vi "AVQ8347 Span Span.vi"(8 "Error In":errorcluster, 9 "Span Unit (nm)":T1(ring)=enum."nm", 10 "Span Value (700)":dbl=700.0 format="%.2f", 11 "VISA Session":refnum<visa-resource-name>) -> (0 "Error Out":errorcluster, 2 "Send Code":string, 3 "Copy VISA Session":refnum<visa-resource-name>)   [LabVIEW 2018]
doc: "Setting of the analysis wavelength span"
panel:
  # "Span Span"
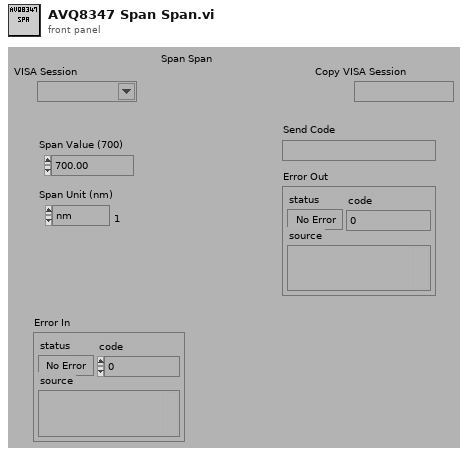
[diagram p1: front panel]
types:
  T1 = enum16{"um", "nm", "nm/DIV", "mm", "THz", "GHz", "THz/DIV", "GHz/DIV"}
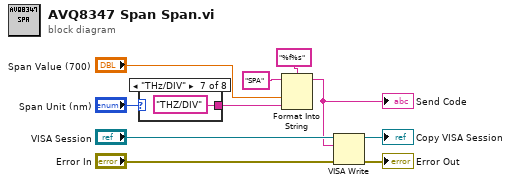
[diagram p0: block diagram]
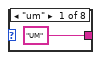
[diagram p2: hidden frame]
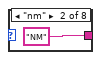
[diagram p3: hidden frame]
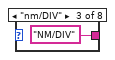
[diagram p4: hidden frame]
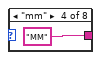
[diagram p5: hidden frame]
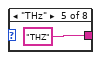
[diagram p6: hidden frame]
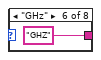
[diagram p7: hidden frame]
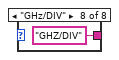
[diagram p8: hidden frame]
diagram:
  n1 = case shown="\"THz/DIV\"" "Span Unit (nm)" {
    tunnel: ["UM" "NM" "NM/DIV" "MM" "THZ" "GHZ" "THZ/DIV" "GHZ/DIV"] -> w1
    frame "um" {
    }
    frame "nm" {
    }
    frame "nm/DIV" {
    }
    frame "mm" {
    }
    frame "THz" {
    }
    frame "GHz" {
    }
    frame "THz/DIV" {
    }
    frame "GHz/DIV" {
    }
  }
  n2 = Format Into String(format string="%f%s", initial string="SPA", "Span Value (700)", w1) -> (resulting string=w2:string)  [unwired: 1 in, 1 out]
  "Send Code" <- w2
  n3 = VISA Write(VISA resource name="VISA Session", write buffer=w2, error in (no error)="Error In") -> (VISA resource name out=→"Copy VISA Session":refnum<visa-resource-name>, error out=→"Error Out":errorcluster)  [unwired: 1 out]
